vi "Get Data I16_32.vi"(8 "error in (no error)":errorcluster, 11 "DAQmx Digitizer in":refnum<class "DAQmx Digitizer.lvclass">) -> (0 "error out":errorcluster, 1 "I32 data out":i32[][](array[numeric]), 2 "data":i16[][](array[numeric]), 3 "DAQmx Digitizer out":refnum<class "DAQmx Digitizer.lvclass">, 4 "Finished":bool, 5 "Current DAQ read position":i32)   [LabVIEW 2021, in "DAQmx Digitizer.lvclass"]
uses:
  DAQmx Digitizer.lvclass
  C:/GitHub/NHMFL_Core/Libraries/Instruments/Pulse Driver/Pulse Driver.lvclass
  C:/GitHub/NHMFL_Core/Libraries/Instruments/Pulse Driver/Lockin Digitizer Driver/Lockin Digitizer Driver.lvclass
  Instruments/Pulse Driver/Pulse Driver.lvclass/Pulse Driver.ctl
  <vilib>/DAQmx/read.llb/DAQmx Read (Analog 2D I16 NChan NSamp).vi
  Instruments/Pulse Driver/Read Current read position.vi
  Instruments/Pulse Driver/Read Samples per channel.vi
  Instruments/Pulse Driver/Read Samples per read.vi
  <vilib>/DAQmx/miscellaneous.llb/DAQmx Fill In Error Info.vi
  DAQmx Digitizer.lvclass/DAQmx Digitizer.ctl
  <resource>/objmgr/daqmx.rc
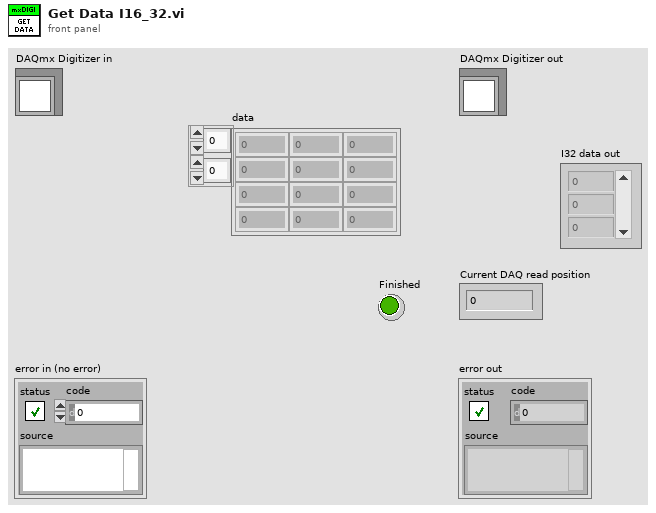
[diagram p1: front panel]
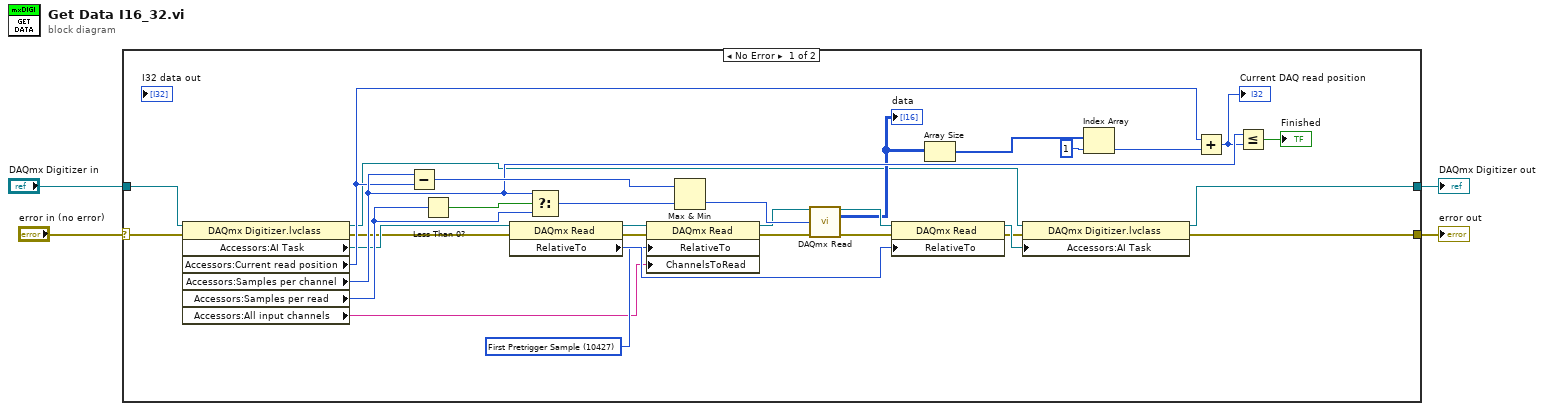
[diagram p0: block diagram]
diagram:
  n1 = case shown="No Error" "error in (no error)" {
    selector: "error in (no error)" -> [w27 w37]
    tunnel: [w14 w37] -> w3
    tunnel: [w17 w36] -> w1
    tunnel: "DAQmx Digitizer in" -> [w35 w36]
    frame No Error {
      w10 = 10427 items=["First Sample"=10424, "Current Read Position"=10425, "Reference Trigger"=10426, "First Pretrigger Sample"=10427, "Most Recent Sample"=10428] ("RelativeTo")
      n2 = property class="DAQmx Digitizer.lvclass"(reference=w35, error in=w27) -> (reference out=w18:refnum<class "DAQmx Digitizer.lvclass">, error out=w12:errorcluster, "Accessors:AI Task"=w13:refnum<k21>, "Accessors:Current read position"=w19:i32, "Accessors:Samples per channel"=w28:i32, "Accessors:Samples per read"=w26:i32, "Accessors:All input channels"=w5:string)
      n3 = Subtract(x=w28, y=w19) -> (x-y=w34:i32)
      n4 = Less Than 0?(x=w26) -> (x < 0?=w30:bool)
      n5 = property class="DAQmx Read"(reference=w13, error in=w12) -> (reference out=w9:refnum<k21>, error out=w8:errorcluster, "RelativeTo"=w11:i32)
      n6 = Select(t=w28, s=w30, f=w26) -> (s? t:f=w29:i32)
      n7 = property class="DAQmx Read"(reference=w9, error in=w8, "RelativeTo"=w10, "ChannelsToRead"=w5) -> (reference out=w6:refnum<k21>, error out=w7:errorcluster)
      n8 = Max & Min(x=w34, y=w29) -> (min(x,y)=w33:i32)  [unwired: 1 out]
      n9 = call-poly <vilib>:"DAQmx Read.vi"("task/channels in"=w6, "number of samples per channel"=w33, "error in"=w7) -> ("task out"=w32:refnum<k21>, "data"=w24:i16[][], "error out"=w31:errorcluster)  [unwired: 1 in, 9 out]
      "data" <- w24
      n10 = property class="DAQmx Read"(reference=w32, error in=w31, "RelativeTo"=w11) -> (reference out=w16:refnum<k21>, error out=w15:errorcluster)
      n11 = Array Size(array=w24) -> (size(s)=w23:i32[])
      n12 = property class="DAQmx Digitizer.lvclass"(reference=w18, error in=w15, "Accessors:AI Task"=w16) -> (reference out=w17:refnum<class "DAQmx Digitizer.lvclass">, error out=w14:errorcluster)
      n13 = Index Array(array=w23, index=1) -> (element=w21:i32)
      n14 = Add(x=w19, y=w21) -> (x+y=w20:i32)
      "Current DAQ read position" <- w20
      n15 = Less Or Equal?(x=w28, y=w20) -> (x <= y?=→"Finished":bool)
    }
    frame Error {
    }
  }
  "error out" <- w3
  "DAQmx Digitizer out" <- w1
